vi "global_var.vi"() -> ()   [LabVIEW 2018]
panel:
  out "flag_press":bool
  out "finished":u32
  out "total box":u32
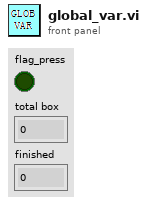
[diagram p1: front panel]
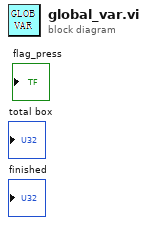
[diagram p0: block diagram]
diagram:
